vi "Resize Array.vi"(6 "Variant in":variant, 7 "Shift Pressed?":bool, 8 "error in (no error)":errorcluster, 10 "QD Combo Box Ref":refnum<vi>, 11 "QD Launch VI Ref":refnum<vi>) -> (0 "error out":errorcluster, 4 "Variant out":variant)   [LabVIEW 2017]
doc: "Resize an array control or indicator. Defaults to the size of the array unless you type a number in the QD box before you hit the shortcut\n\nDefault Shortcut - [L]"
panel:
  in  "Undo Name":string="Reset to Origin"
  # "Do not change the connector pane of this VI.\n\nSee the block diagram for directions on how to use this template."
  # "Specify the name of the Undo transaction"
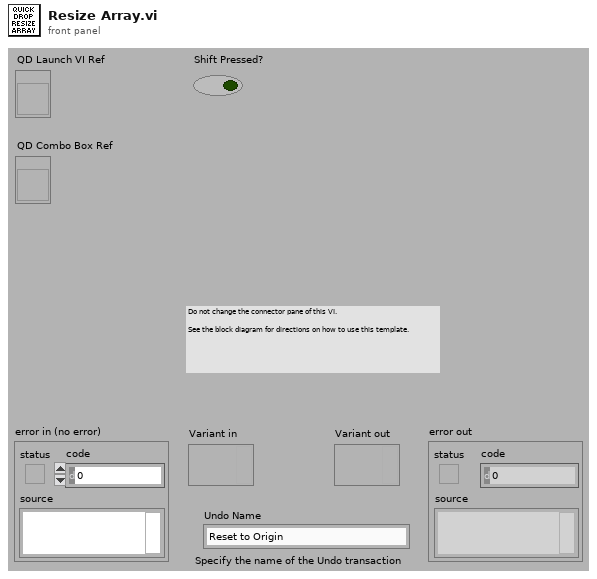
[diagram p1: front panel]
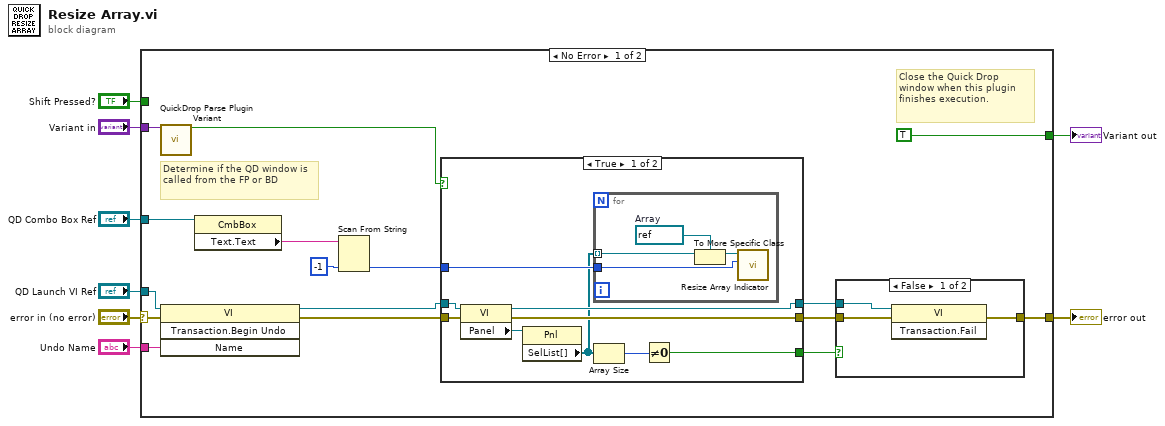
[diagram p0: block diagram]
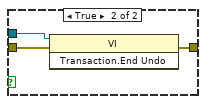
[diagram p2: hidden frame]
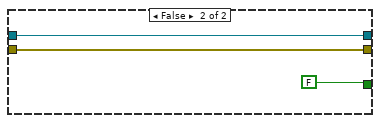
[diagram p3: hidden frame]
diagram:
  n1 = case shown="No Error" "error in (no error)" {
    selector: "error in (no error)" -> [w23 w47]
    tunnel: [w17 w47] -> w7
    tunnel: "QD Launch VI Ref" -> [w22 _]
    tunnel: "Shift Pressed?" -> [_ _]
    tunnel: "QD Combo Box Ref" -> [w15 _]
    tunnel: "Variant in" -> [w24 _]
    tunnel: "Undo Name" -> [w21 _]
    tunnel: [TRUE _] -> w1
    frame No Error {
      # "Close the Quick Drop window when this plugin finishes execution."
      # "Determine if the QD window is called from the FP or BD"
      n2 = call <vilib>:"QuickDrop Parse Plugin Variant.vi"("QDKS Variant in"=w24) -> ("QD Launch VI Panel?"=w19:bool)  [unwired: 12 in, 2 out]
      n3 = invoke class="VI" method="Transaction.Begin Undo"(reference=w22, error in=w23, "Name"=w21) -> (reference out=w16:refnum<vi>, error out=w18:errorcluster)  [unwired: 1 in, 2 out]
      n4 = property class="CmbBox"(reference=w15) -> ("Text.Text"=w14:string)  [unwired: 1 in, 2 out]
      n5 = Scan From String(input string=w14, default 1=-1 ("Max Rows (-1)")) -> (output 1=w12:i32)  [unwired: 3 in, 3 out]
      n6 = case shown="True" w19 {
        tunnel: w18 -> [w35 w44]
        tunnel: w16 -> [w39 w45]
        tunnel: w12 -> [w37 _]
        tunnel: [w36 w45] -> w11
        tunnel: [w34 w44] -> w10
        tunnel: [w31 FALSE] -> w9
        frame True {
          n7 = property class="VI"(reference=w39, error in=w35) -> (reference out=w36:refnum<vi>, error out=w34:errorcluster, "Panel"=w38:refnum<vi>)
          n8 = property class="Pnl"(reference=w38) -> ("SelList[]"=w33:refnum<vi>[])  [unwired: 1 in, 2 out]
          n9 = for {
            tunnel: w33 -> [w43] mode=indexing
            tunnel: w37 -> [w40]
            w42 = refnum<vi> refnum  # Array
            n10 = To More Specific Class(target class=w42, reference=w43) -> (specific class reference=w41:refnum<vi>)  [unwired: 1 in, 1 out]
            n11 = call "Resize Array Indicator.vi"("Max Rows (-1)"=w40, "Arr Refnum"=w41) -> ()  [unwired: 10 in]
          }
          n12 = Array Size(array=w33) -> (size(s)=w32:i32)
          n13 = Not Equal To 0?(x=w32) -> (x != 0?=w31:bool)
        }
        frame False {
        }
      }
      n14 = case shown="False" w9 {
        tunnel: [w25 w30] -> w17
        tunnel: w11 -> [w27 w29]
        tunnel: w10 -> [w26 w28]
        frame False {
          n15 = invoke class="VI" method="Transaction.Fail"(reference=w27, error in=w26) -> (error out=w25:errorcluster)  [unwired: 1 in, 2 out]
        }
        frame True {
          n16 = invoke class="VI" method="Transaction.End Undo"(reference=w29, error in=w28) -> (error out=w30:errorcluster)  [unwired: 1 in, 2 out]
        }
      }
    }
    frame Error {
    }
  }
  "error out" <- w7
  "Variant out" <- w1
